vi "HighSpeedAverage8.vi"(0 "x 1":fxp<+/-,16,14>, 1 "x 5":fxp<+/-,16,14>, 2 "x 6":fxp<+/-,16,14>, 5 "x 2":fxp<+/-,16,14>, 7 "x 3":fxp<+/-,16,14>, 9 "x 4":fxp<+/-,16,14>, 11 "input valid":bool=TRUE, 12 "x 7":fxp<+/-,16,14>, 13 "x 8":fxp<+/-,16,14>) -> (4 "average":fxp<+/-,16,14>, 15 "output valid":bool)   [LabVIEW 2013]
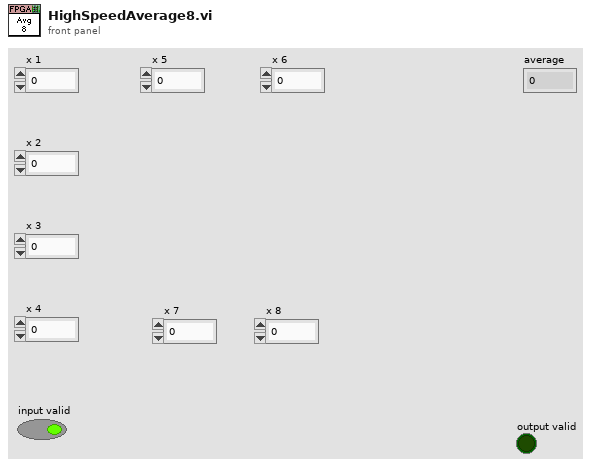
[diagram p1: front panel]
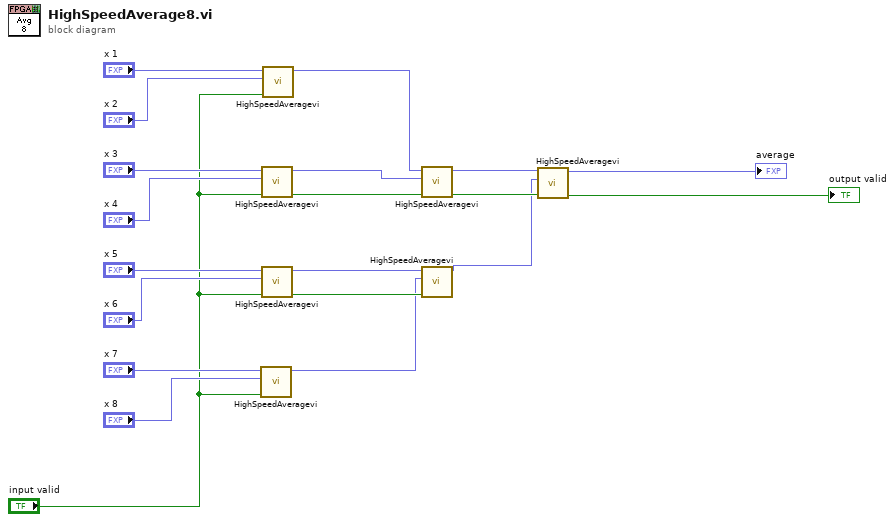
[diagram p0: block diagram]
diagram:
  n1 = call "HighSpeedAveragevi.vi"("input valid"="input valid", "y"="x 8", "x"="x 7") -> ("(x+y)/2"=w6:fxp<+/-,16,14>)  [unwired: 7 in, 1 out]
  n2 = call "HighSpeedAveragevi.vi"("input valid"="input valid", "y"="x 4", "x"="x 3") -> ("output valid"=w10:bool, "(x+y)/2"=w9:fxp<+/-,16,14>)  [unwired: 7 in]
  n3 = call "HighSpeedAveragevi.vi"("input valid"="input valid", "y"="x 6", "x"="x 5") -> ("output valid"=w8:bool, "(x+y)/2"=w7:fxp<+/-,16,14>)  [unwired: 7 in]
  n4 = call "HighSpeedAveragevi.vi"("input valid"="input valid", "y"="x 2", "x"="x 1") -> ("(x+y)/2"=w11:fxp<+/-,16,14>)  [unwired: 7 in, 1 out]
  n5 = call "HighSpeedAveragevi.vi"("input valid"=w10, "y"=w9, "x"=w11) -> ("output valid"=w4:bool, "(x+y)/2"=w5:fxp<+/-,16,14>)  [unwired: 7 in]
  n6 = call "HighSpeedAveragevi.vi"("input valid"=w8, "y"=w6, "x"=w7) -> ("(x+y)/2"=w3:fxp<+/-,16,14>)  [unwired: 7 in, 1 out]
  n7 = call "HighSpeedAveragevi.vi"("input valid"=w4, "y"=w3, "x"=w5) -> ("output valid"=→"output valid":bool, "(x+y)/2"=→"average":fxp<+/-,16,14>)  [unwired: 7 in]
